vi "Select Fabric Style.vi"(1 "connectString":string, 2 "Vendor":string) -> (0 "fabStyles":string[](array[string]))   [LabVIEW 2012]
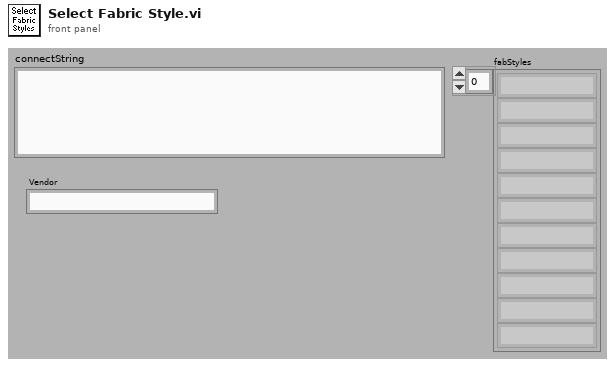
[diagram p1: front panel]
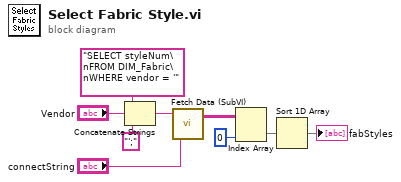
[diagram p0: block diagram]
diagram:
  n1 = Concatenate Strings("SELECT styleNum\nFROM DIM_Fabric\nWHERE vendor = '", "Vendor", "';" ("string")) -> (w5:string)
  n2 = call "Fetch Data (SubVI).vi"("connectString"="connectString", "query string"=w5) -> ("recordset data"=w9:string[][])  [unwired: 1 in, 1 out]
  n3 = Index Array(array=w9, index (col)=0 ("disabled index (col)")) -> (element=w2:string[])  [unwired: 1 in]
  n4 = Sort 1D Array(array=w2) -> (sorted array=→"fabStyles":string[])
